vi "ActionVIOnLoad.vi"(8 "error in (no error)":errorcluster, 11 "Device Item Ref In":T1 format="%.0x") -> (0 "error out":errorcluster, 3 "Device Item Ref out":T1 format="%.0x")   [LabVIEW 2020, in "G5 Regatron Custom Device System Explorer.lvlib"]
uses:
  G5 Regatron Custom Device System Explorer.lvlib
  <vilib>/NI VeriStand/Custom Device API/Custom Device Item Ref.ctl
  <vilib>/NI VeriStand/Custom Device API/Custom Device API.lvlib
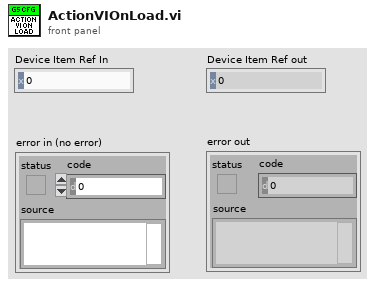
[diagram p1: front panel]
types:
  T1 = typedef "Custom Device API.lvlib/Custom Device Item Ref.ctl" = u64
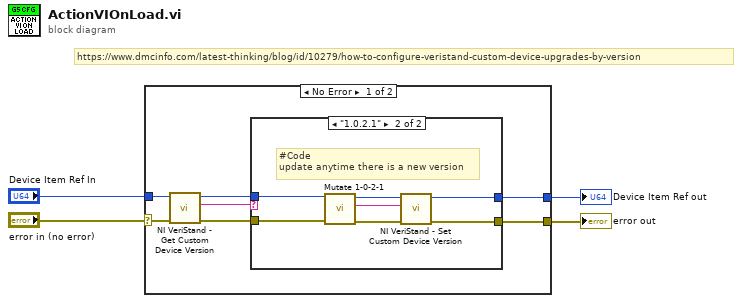
[diagram p0: block diagram]
diagram:
  # "https://www.dmcinfo.com/latest-thinking/blog/id/10279/how-to-configure-veristand-custom-device-upgrades-by-version"
  n1 = case shown="No Error" "error in (no error)" {
    selector: "error in (no error)" -> [w10 w22]
    tunnel: "Device Item Ref In" -> [w11 w21]
    tunnel: [w6 w22] -> w3
    tunnel: [w5 w21] -> w2
    frame No Error {
      n2 = call <vilib>:"NI VeriStand - Get Custom Device Version.vi"("error in (no error)"=w10, "Device Ref in"=w11) -> ("error out"=w8:errorcluster, "Value"=w9:string, "Device Ref out"=w7:T1)  [unwired: 7 in]
      n3 = case shown="\"1.0.2.1\"" w9 {
        tunnel: w8 -> [w12 w20]
        tunnel: w7 -> [w13 w19]
        tunnel: [w12 w15] -> w6
        tunnel: [w13 w14] -> w5
        frame "False", Default {
        }
        frame "1.0.2.1" {
          # "#Code\nupdate anytime there is a new version"
          n4 = call "Mutate 1-0-2-1.vi"("error in (no error)"=w20, "Device Ref in"=w19) -> ("error out"=w18:errorcluster, "New CD Version"=w16:string, "Device Ref out"=w17:T1)  [unwired: 7 in]
          n5 = call <vilib>:"NI VeriStand - Set Custom Device Version.vi"("error in (no error)"=w18, "Value"=w16, "Device Ref in"=w17) -> ("error out"=w15:errorcluster, "Device Ref out"=w14:T1)  [unwired: 7 in]
        }
      }
    }
    frame Error {
    }
  }
  "error out" <- w3
  "Device Item Ref out" <- w2
